vi "P Term.vi"(7 "Output Range":T1={"Min"=-50.0, "Max"=50.0}, 9 "Error":dbl, 10 "P Band":dbl=0.05) -> (2 "Output":dbl, 5 "Remaining Range":T1)   [LabVIEW 2020, in "IG PID.lvlib" / "PID.lvclass"]
uses:
  PID.lvclass
  Output Range.ctl
  IG PID.lvlib
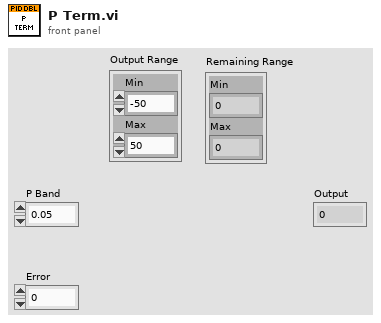
[diagram p1: front panel]
types:
  T1 = typedef "IG PID.lvlib/Output Range.ctl" = cluster{"Min":dbl, "Max":dbl}
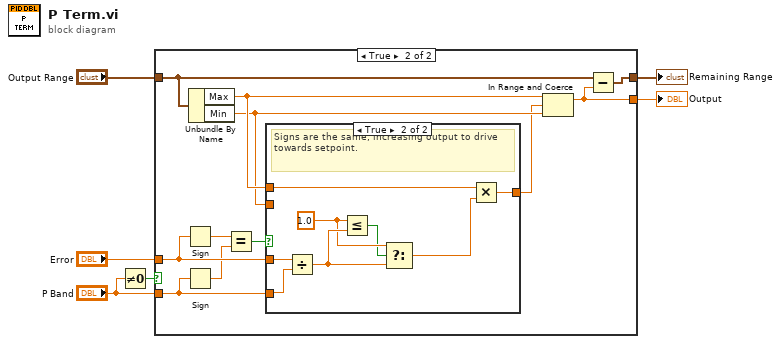
[diagram p0: block diagram]
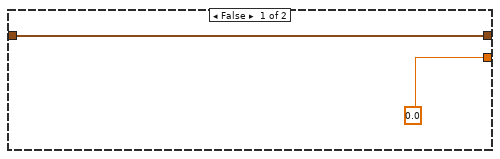
[diagram p2: hidden frame]
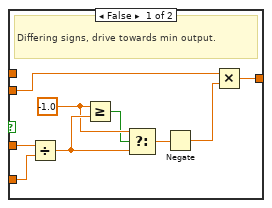
[diagram p3: hidden frame]
diagram:
  n1 = Not Equal To 0?(x="P Band") -> (x != 0?=w1:bool)
  n2 = case shown="True" w1 {
    tunnel: "Error" -> [_ w19]
    tunnel: "Output Range" -> [w8 w15]
    tunnel: [0.0 w9] -> w4
    tunnel: [w8 w14] -> w3
    tunnel: "P Band" -> [_ w13]
    frame False {
    }
    frame True {
      n3 = Sign(1:w19) -> (0:w18:dbl)
      n4 = Sign(1:w13) -> (0:w17:dbl)
      n5 = Unbundle By Name(w15) -> ("Max"=w12:dbl, "Min"=w11:dbl)
      n6 = Equal?(x=w18, y=w17) -> (x = y?=w16:bool)
      n7 = case shown="True" w16 {
        tunnel: w19 -> [w25 w36]
        tunnel: w13 -> [w24 w35]
        tunnel: w11 -> [w23 _]
        tunnel: w12 -> [_ w32]
        tunnel: [w21 w29] -> w10
        frame False {
          w27 = -1.0 ("y")
          # "Differing signs, drive towards min output."
          n8 = Divide(x=w25, y=w24) -> (x/y=w28:dbl)
          n9 = Greater Or Equal?(x=w27, y=w28) -> (x >= y?=w22:bool)
          n10 = Select(t=w27, s=w22, f=w28) -> (s? t:f=w26:dbl)
          n11 = Negate(x=w26) -> (-x=w20:dbl)
          n12 = Multiply(x=w23, y=w20) -> (x*y=w21:dbl)
        }
        frame True {
          w33 = 1.0 ("y")
          # "Signs are the same, increasing output to drive towards setpoint."
          n13 = Divide(x=w36, y=w35) -> (x/y=w34:dbl)
          n14 = Less Or Equal?(x=w33, y=w34) -> (x <= y?=w30:bool)
          n15 = Select(t=w33, s=w30, f=w34) -> (s? t:f=w31:dbl)
          n16 = Multiply(x=w32, y=w31) -> (x*y=w29:dbl)
        }
      }
      n17 = In Range and Coerce(upper limit=w12, x=w10, lower limit=w11) -> (coerced(x)=w9:dbl)  [unwired: 1 out]
      n18 = Subtract(x=w15, y=w9) -> (x-y=w14:T1)
    }
  }
  "Output" <- w4
  "Remaining Range" <- w3
